vi "Engine Out - Diesel - EGR Actuation.vi"(10 "LowP EGR Position Setpoint [%Open]":sgl, 11 "HighP EGR Position Setpoint [%Open]":sgl) -> (2 "Throttle Channel2 DC [%]":sgl, 3 "Throttle Channel1 Setpoint [%Open]":sgl)   [LabVIEW 2015, in "ECS-RT.lvlib"]
uses:
  ECS-RT.lvlib
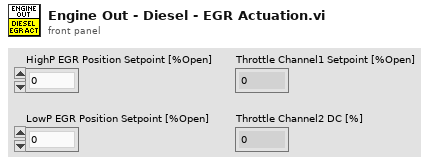
[diagram p1: front panel]
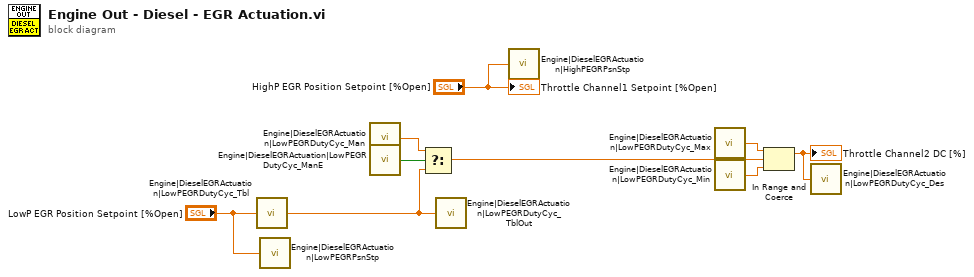
[diagram p0: block diagram]
diagram:
  n1 = call "Engine|DieselEGRActuation|LowPEGRDutyCyc_Tbl"("X Index"="LowP EGR Position Setpoint [%Open]") -> ("Y"=w2:sgl)
  n2 = call "Engine|DieselEGRActuation|LowPEGRPsnStp"("Value"="LowP EGR Position Setpoint [%Open]") -> ()
  n3 = call "Engine|DieselEGRActuation|LowPEGRDutyCyc_Man"() -> ("Value"=w5:sgl)
  n4 = call "Engine|DieselEGRActuation|LowPEGRDutyCyc_ManE"() -> ("Value"=w6:bool)
  n5 = Select(t=w5, s=w6, f=w2) -> (s? t:f=w7:sgl)
  n6 = call "Engine|DieselEGRActuation|LowPEGRDutyCyc_TblOut"("Value"=w2) -> ()
  n7 = call "Engine|DieselEGRActuation|HighPEGRPsnStp"("Value"="HighP EGR Position Setpoint [%Open]") -> ()
  n8 = call "Engine|DieselEGRActuation|LowPEGRDutyCyc_Max"() -> ("Value"=w8:sgl)
  n9 = call "Engine|DieselEGRActuation|LowPEGRDutyCyc_Min"() -> ("Value"=w9:sgl)
  n10 = In Range and Coerce(upper limit=w8, x=w7, lower limit=w9) -> (coerced(x)=w1:sgl)  [unwired: 1 out]
  "Throttle Channel2 DC [%]" <- w1
  n11 = call "Engine|DieselEGRActuation|LowPEGRDutyCyc_Des"("Value"=w1) -> ()
  "Throttle Channel1 Setpoint [%Open]" <- "HighP EGR Position Setpoint [%Open]"
